vi "DAQ_SynchrStartSub.vi"(1 "DAQ_AI_task_out":refnum<k21>, 2 "counter_task_out":refnum<k21>[](array[refnum]), 5 "error in":errorcluster caption="error out") -> (19 "error out":errorcluster caption="错误输出")   [LabVIEW 2020, in "NI_DAQ.lvclass"]
uses:
  NI_DAQ.lvclass
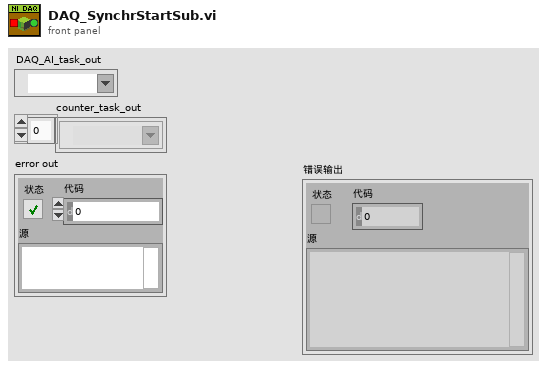
[diagram p1: front panel]
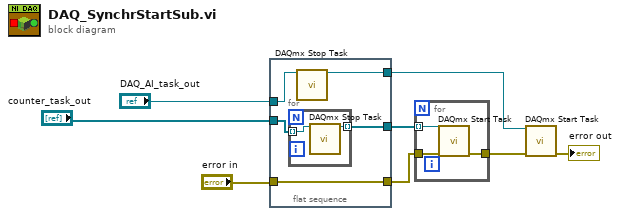
[diagram p0: block diagram]
diagram:
  n1 = flat-sequence {
    tunnel: "DAQ_AI_task_out" -> [w12]
    tunnel: "counter_task_out" -> [w13]
    tunnel: [w11] -> w7
    tunnel: [w10] -> w6
    tunnel: [w9] -> w3
    tunnel: "error in" -> [w9]
    frame #0 {
      n2 = for {
        tunnel: w13 -> [w15] mode=indexing
        tunnel: [w14] -> w11 mode=indexing
        n3 = call <vilib>:"DAQmx Stop Task.vi"("task/channels in"=w15) -> ("task out"=w14:refnum<k21>)  [unwired: 13 in, 1 out]
      }
      n4 = call <vilib>:"DAQmx Stop Task.vi"("task/channels in"=w12) -> ("task out"=w10:refnum<k21>)  [unwired: 13 in, 1 out]
    }
  }
  n5 = for {
    tunnel: w3 -> [w18]
    tunnel: [w17] -> w8
    tunnel: w7 -> [w16] mode=indexing
    n6 = call <vilib>:"DAQmx Start Task.vi"("task/channels in"=w16, "error in"=w18) -> ("error out"=w17:errorcluster)  [unwired: 12 in, 1 out]
  }
  n7 = call <vilib>:"DAQmx Start Task.vi"("task/channels in"=w6, "error in"=w8) -> ("error out"=→"error out":errorcluster)  [unwired: 12 in, 1 out]
